vi "digital galvo position ver2.vi"(8 "error in":errorcluster) -> (0 "error out":errorcluster)   [LabVIEW 2015]
uses:
  <vilib>/DAQmx/write.llb/DAQmx Write (Digital 1D U32 1Chan NSamp).vi
  <vilib>/DAQmx/create/channels.llb/DAQmx Create Channel (DO-Digital Output).vi
  <vilib>/DAQmx/configure/timing.llb/DAQmx Timing (Sample Clock).vi
  <vilib>/DAQmx/create/channels.llb/DAQmx Create Channel (CO-Pulse Generation-Frequency).vi
  <vilib>/DAQmx/configure/timing.llb/DAQmx Timing (Implicit).vi
  <vilib>/DAQmx/miscellaneous.llb/DAQmx Fill In Error Info.vi
  <resource>/objmgr/daqmx.rc
panel:
  out "array":u32[](array[numeric])
  out "appended array":bool[][](array[boolean])
  in  "initial x":u16=31800
  in  "initial y":u16=42800
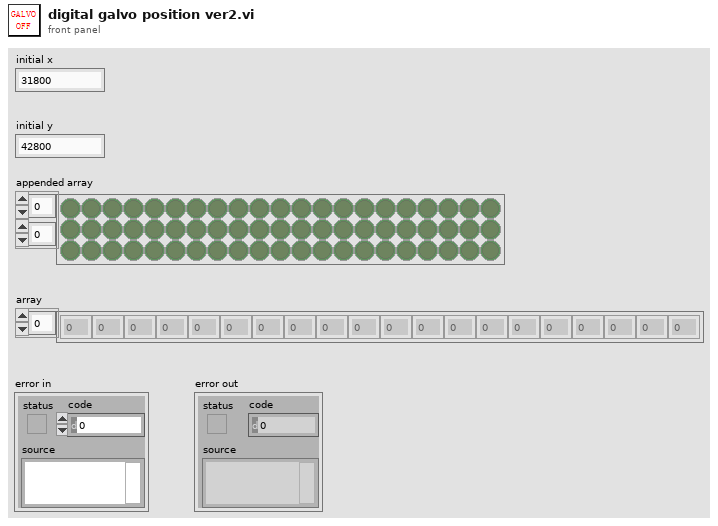
[diagram p1: front panel]
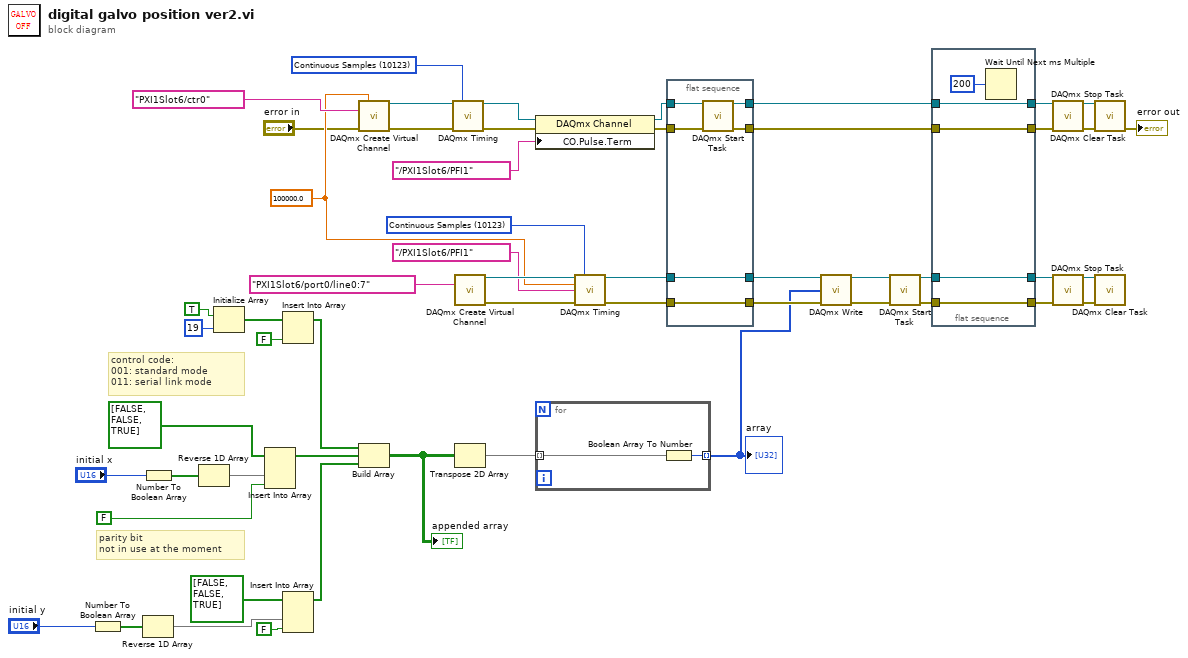
[diagram p0: block diagram]
diagram:
  w43 = 10123 items=["Finite Samples"=10178, "Continuous Samples"=10123, "Hardware Timed Single Point"=12522] ("sample mode")
  w44 = 100000.0 ("frequency")
  w49 = 10123 items=["Finite Samples"=10178, "Continuous Samples"=10123, "Hardware Timed Single Point"=12522] ("sample mode")
  # "parity bit\nnot in use at the moment"
  # "control code:\n001: standard mode\n011: serial link mode"
  n1 = Number To Boolean Array(number="initial y") -> (Boolean array=w29:bool[])
  n2 = Reverse 1D Array(array=w29) -> (reversed array=w27:bool[])
  n3 = Number To Boolean Array(number="initial x") -> (Boolean array=w20:bool[])
  n4 = Reverse 1D Array(array=w20) -> (reversed array=w18:bool[])
  n5 = Initialize Array(TRUE ("element"), 19 ("dimension size")) -> (w23:bool[])
  n6 = Insert Into Array(array=bool[] [FALSE, FALSE, TRUE] ("Array"), new element #1=w18, new element #2=FALSE) -> (w16:bool[])  [unwired: 1 in]
  n7 = Insert Into Array(array=w23, new element=FALSE ("element")) -> (w22:bool[])  [unwired: 1 in]
  n8 = Insert Into Array(array=bool[] [FALSE, FALSE, TRUE] ("Array"), new element #1=w27, new element #2=FALSE) -> (w15:bool[])  [unwired: 1 in]
  n9 = call-poly <vilib>:"DAQmx Create Virtual Channel.vi"("frequency"=w44, "counter"=tag "PXI1Slot6/ctr0", "error in"="error in") -> ("task out"=w54:refnum<k21>, "error out"=w53:errorcluster)  [unwired: 11 in]
  n10 = Build Array(w22, w16, w15) -> (w14:bool[][])
  "appended array" <- w14
  n11 = call-poly <vilib>:"DAQmx Timing.vi"("task/channels in"=w54, "sample mode"=w49, "error in"=w53) -> ("task out"=w52:refnum<k21>, "error out"=w51:errorcluster)  [unwired: 11 in]
  n12 = call-poly <vilib>:"DAQmx Create Virtual Channel.vi"("lines"=tag "PXI1Slot6/port0/line0:7") -> ("task out"=w48:refnum<k21>, "error out"=w47:errorcluster)  [unwired: 13 in]
  n13 = Transpose 2D Array(2D array=w14) -> (transposed array=w13:bool[][])
  n14 = property class="DAQmx Channel"(reference=w52, error in=w51, "CO.Pulse.Term"=tag "/PXI1Slot6/PFI1") -> (reference out=w42:refnum<k21>, error out=w41:errorcluster)
  n15 = for {
    tunnel: w13 -> [w57] mode=indexing
    tunnel: [w56] -> w12 mode=indexing
    n16 = Boolean Array To Number(Boolean array=w57) -> (number=w56:u32)
  }
  "array" <- w12
  n17 = call-poly <vilib>:"DAQmx Timing.vi"("task/channels in"=w48, "sample mode"=w43, "rate"=w44, "source"=tag "/PXI1Slot6/PFI1", "error in"=w47) -> ("task out"=w40:refnum<k21>, "error out"=w39:errorcluster)  [unwired: 9 in]
  n18 = flat-sequence {
    tunnel: w42 -> [w63]
    tunnel: w41 -> [w62]
    tunnel: w40 -> [w58]
    tunnel: [w61] -> w37
    tunnel: w39 -> [w61]
    tunnel: [w60] -> w6
    tunnel: [w59] -> w3
    tunnel: [w58] -> w38
    frame #0 {
      n19 = call <vilib>:"DAQmx Start Task.vi"("task/channels in"=w63, "error in"=w62) -> ("task out"=w60:refnum<k21>, "error out"=w59:errorcluster)  [unwired: 12 in]
    }
  }
  n20 = call-poly <vilib>:"DAQmx Write.vi"("task/channels in"=w38, "data"=w12, "error in"=w37) -> ("task out"=w36:refnum<k21>, "error out"=w35:errorcluster)  [unwired: 10 in, 1 out]
  n21 = call <vilib>:"DAQmx Start Task.vi"("task/channels in"=w36, "error in"=w35) -> ("task out"=w10:refnum<k21>, "error out"=w8:errorcluster)  [unwired: 12 in]
  n22 = flat-sequence {
    tunnel: [w67] -> w9
    tunnel: w10 -> [w67]
    tunnel: w8 -> [w66]
    tunnel: [w66] -> w7
    tunnel: w6 -> [w65]
    tunnel: [w65] -> w5
    tunnel: [w64] -> w4
    tunnel: w3 -> [w64]
    frame #0 {
      n23 = Wait Until Next ms Multiple(millisecond multiple=u32 200) -> ()  [unwired: 1 out]
    }
  }
  n24 = call <vilib>:"DAQmx Stop Task.vi"("task/channels in"=w5, "error in"=w4) -> ("task out"=w33:refnum<k21>, "error out"=w34:errorcluster)  [unwired: 12 in]
  n25 = call <vilib>:"DAQmx Stop Task.vi"("task/channels in"=w9, "error in"=w7) -> ("task out"=w31:refnum<k21>, "error out"=w32:errorcluster)  [unwired: 12 in]
  n26 = call <vilib>:"DAQmx Clear Task.vi"("task in"=w33, "error in"=w34) -> ("error out"=→"error out":errorcluster)  [unwired: 13 in]
  n27 = call <vilib>:"DAQmx Clear Task.vi"("task in"=w31, "error in"=w32) -> ()  [unwired: 13 in, 1 out]
